vi "SaveGestureCommon.vi"(8 "error in (no error)":errorcluster, 11 ".NET Refnum in":refnum<k24>) -> (0 "error out":errorcluster, 2 "Gesture Common":T1, 3 ".NET Refnum Passthrough":refnum<k24>)   [LabVIEW 2011, in "LVH-Leap.lvlib"]
uses:
  LVH-Leap.lvlib
  Type Defs/Gesture Common.ctl
  Type Defs/Gesture Type.ctl
  Type Defs/Gesture State.ctl
  C:/github/labviewhacker/LVH-Leap/LabVIEW/vi.lib/LabVIEW Hacker/Leap/Private/Libs/LeapCSharp.NET3.5.dll
  Libs/LeapCSharp.NET3.5.dll
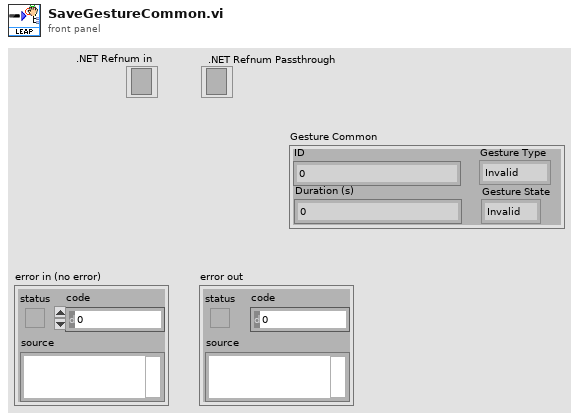
[diagram p1: front panel]
types:
  T1 = typedef "LVH-Leap.lvlib/Gesture Common.ctl" = cluster{"ID":i32, "Duration (s)":dbl, "Gesture Type":T2, "Gesture State":T3}
  T2 = typedef "LVH-Leap.lvlib/Gesture Type.ctl" = enum16{"Invalid", "Swipe", "Circle", "Screen Tap", "Key Tap"}
  T3 = typedef "LVH-Leap.lvlib/Gesture State.ctl" = enum16{"Invalid", "Start", "Update", "Stop"}
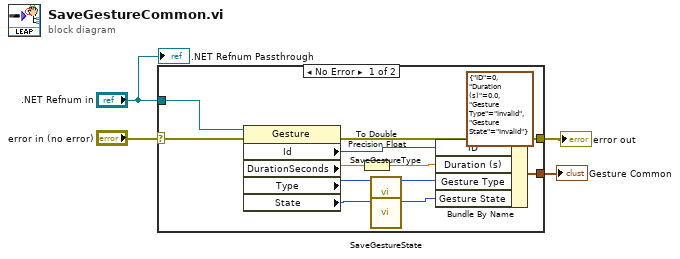
[diagram p0: block diagram]
diagram:
  n1 = case shown="No Error" "error in (no error)" {
    selector: "error in (no error)" -> [w12 w17]
    tunnel: [w16 w17] -> w4
    tunnel: [w14 _] -> w3
    tunnel: ".NET Refnum in" -> [w9 _]
    frame No Error {
      n2 = property class="Gesture"(reference=w9, error in=w12) -> (error out=w16:errorcluster, "Id"=w13:i32, "DurationSeconds"=w7:sgl, "Type"=w6:i32, "State"=w5:i32)  [unwired: 1 out]
      n3 = To Double Precision Float(number=w7) -> (double precision float=w8:dbl)
      n4 = call "SaveGestureType.vi"("Type"=w6) -> ("gesture type"=w10:T2)  [unwired: 10 in]
      n5 = call "SaveGestureState.vi"("State"=w5) -> ("gesture state"=w11:T3)  [unwired: 10 in]
      n6 = Bundle By Name(cluster=T1 {"ID"=0, "Duration (s)"=0.0, "Gesture Type"=enum."Invalid", "Gesture State"=enum."Invalid"} ("Gesture"), "ID"=w13, "Duration (s)"=w8, "Gesture Type"=w10, "Gesture State"=w11) -> (w14:T1)
    }
    frame Error {
    }
  }
  "error out" <- w4
  "Gesture Common" <- w3
  ".NET Refnum Passthrough" <- ".NET Refnum in"
